vi "Asynchronous Engine.vi"(8 "error in":errorcluster, 9 "Parameters":T1, 10 "Parent":string) -> ()   [LabVIEW 2014, in "Waveform-Processing-Custom-Device Engine.lvlib"]
uses:
  Waveform-Processing-Custom-Device Engine.lvlib
  Types/Async Parameters.ctl
  Types/Async FIFOs.ctl
  <vilib>/NI Veristand/Custom Device Waveform API/Single Waveform Read (DBL)/Single Waveform Read (DBL).lvclass
  <userlib>/Circular Buffer/Controls/Circular Buffer Operations.ctl
  <userlib>/Circular Buffer/Instance VIs/Circular Buffer(2D DBL).vi
  Userlib/Error Handling API/Error Handling API.lvlib
  Userlib/Inline Async API/Inline Async API.lvlib
  <userlib>/Circular Buffer/Circular Buffer.lvlib
panel:
  out "Processing Engine Loop Rate (ms)":u32
  out "Tag Results":dbl[](array[numeric])
  in  "Stop":bool
  in  "Samples to average":i32=512
  out "error out":errorcluster
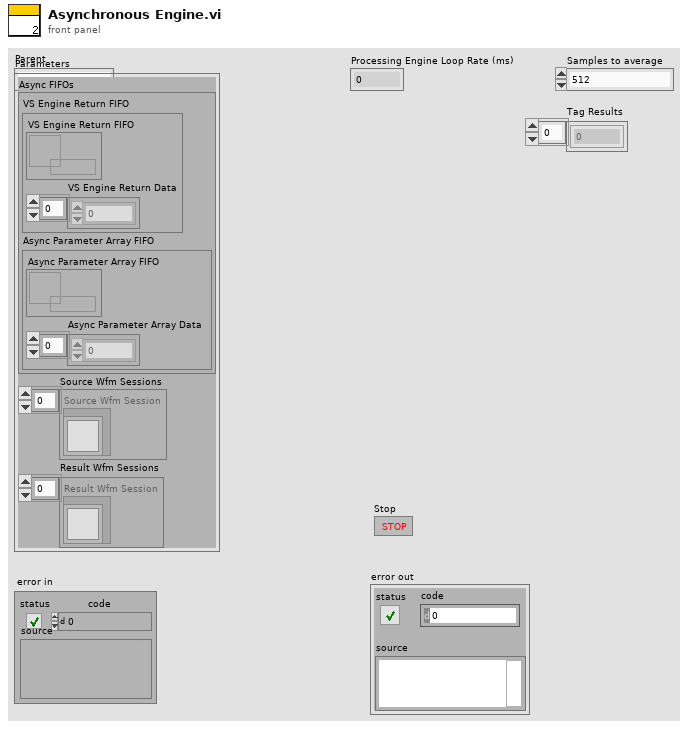
[diagram p1: front panel]
types:
  T1 = typedef "Waveform-Processing-Custom-Device Engine.lvlib/Async Parameters.ctl" = cluster{"Async FIFOs":T2, "Source Wfm Sessions":refnum<class "Single Waveform Read (DBL).lvclass">[], "Result Wfm Sessions":refnum<class "Single Waveform Read (DBL).lvclass">[]}
  T2 = typedef "Waveform-Processing-Custom-Device Engine.lvlib/Async FIFOs.ctl" = cluster{"VS Engine Return FIFO":cluster{"VS Engine Return FIFO":refnum<k33>, "VS Engine Return Data":dbl[]}, "Async Parameter Array FIFO":cluster{"Async Parameter Array FIFO":refnum<k33>, "Async Parameter Array Data":dbl[]}}
  T3 = cluster{"Samples per Channel":u32, "Channels":u32}
  T4 = typedef "Circular Buffer.lvlib/Circular Buffer Operations.ctl" = enum16{"Initialize", "Get Backlog", "Write", "Read (continuous)", "Read (most recent)"}
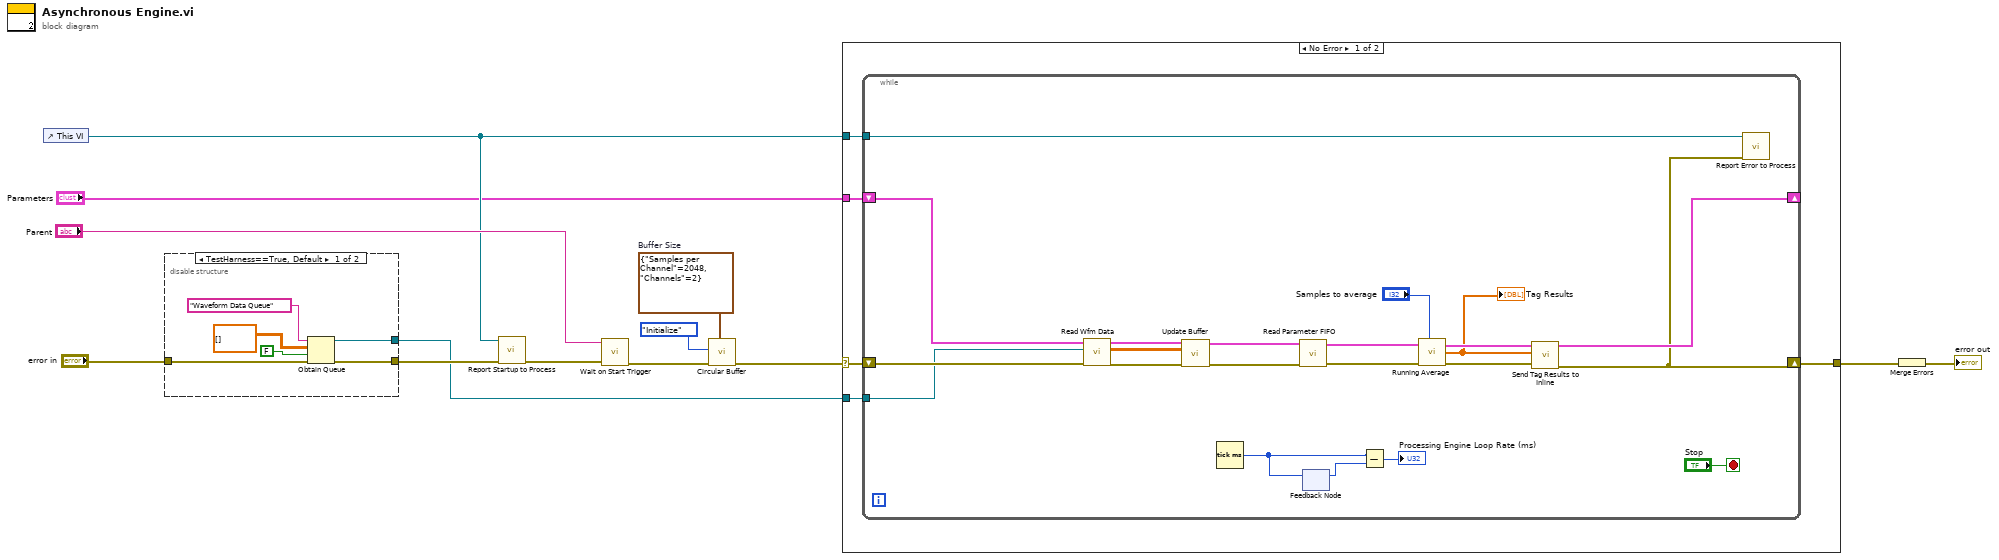
[diagram p0: block diagram]
diagram:
  w3 = T3 {"Samples per Channel"=2048, "Channels"=2}  # Buffer Size
  n1 = control-ref of="This VI"() -> (w11:refnum<vi>)
  n2 = disable-structure shown="TestHarness==True, Default" {
    disable-tunnel: [w16 _] -> w2
    disable-tunnel: [w15 _] -> w7
    disable-tunnel: "error in" -> [w14 _]
    frame condition #0 (active) {
      n3 = Obtain Queue(name (unnamed)="Waveform Data Queue", element data type=dbl[][] [], create if not found? (T)=FALSE, error in (no error)=w14) -> (queue out=w16:refnum<queue>, error out=w15:errorcluster)  [unwired: 1 in, 1 out]
    }
    frame condition #1 {
    }
  }
  n4 = call "Report Startup to Process.vi"("Error"=w7, "This VI"=w11) -> ("error out"=w13:errorcluster)  [unwired: 9 in]
  n5 = call "Wait on Start Trigger.vi"("error in (no error)"=w13, "Name"="Parent") -> ("error out"=w5:errorcluster)  [unwired: 8 in, 1 out]
  n6 = call-poly <userlib>:"Circular Buffer.vi"("Buffer Size"=w3, "error in (no error)"=w5, "Operation"=Circular_Buffer_Operations."Initialize") -> ("error out"=w4:errorcluster)  [unwired: 5 in, 3 out]
  n7 = case shown="No Error" w4 {
    selector: w4 -> [w24 _]
    tunnel: w11 -> [w23 _]
    tunnel: [w22 _] -> w10
    tunnel: w2 -> [w21 _]
    tunnel: "Parameters" -> [w20 _]
    frame No Error {
      n8 = while {
        shift-right: [w28] -> w22
        shift-left: w24 -> [w45]
        tunnel: w23 -> [w44]
        tunnel: w21 -> [w41]
        shift-right: [w29] -> _
        shift-left: w20 -> [w30]
        stop <- "Stop" stop-if-true
        n9 = call "Read Wfm Data.vi"("error in (no error)"=w45, "Queue in"=w41, "Parameters in"=w30) -> ("error out"=w38:errorcluster, "Wfm Data"=w36:dbl[][], "Parameters out"=w40:T1)  [unwired: 6 in]
        n10 = call "Update Buffer.vi"("Error in"=w38, "Wfm data"=w36, "Parameters"=w40) -> ("Error out"=w37:errorcluster, "Parameters dup"=w39:T1)  [unwired: 7 in]
        n11 = Tick Count (ms)() -> (millisecond timer value=w27:u32)
        n12 = call "Read Parameter FIFO.vi"("Error In"=w37, "Parameters in"=w39) -> ("Error Out"=w35:errorcluster, "Parameters out"=w34:T1)  [unwired: 8 in]
        n13 = feedback-in #1(w27) -> ()
        n14 = feedback #1() -> (w26:u32)  [unwired: 1 in]
        n15 = Subtract(x=w27, y=w26) -> (x-y=→"Processing Engine Loop Rate (ms)":u32)
        n16 = call "Running Average.vi"("Samples to average"="Samples to average", "Error In"=w35, "Parameters"=w34) -> ("Error Out"=w32:errorcluster, "Tag Results"=w31:dbl[], "Parameters dup"=w33:T1)  [unwired: 6 in]
        "Tag Results" <- w31
        n17 = call "Send Tag Results to Inline.vi"("Error in"=w32, "Tag Results"=w31, "Parameters"=w33) -> ("Error out"=w28:errorcluster, "Parameters dup"=w29:T1)  [unwired: 7 in]
        n18 = call "Report Error to Process.vi"("Error"=w28, "This VI"=w44) -> ()  [unwired: 10 in]
      }
    }
    frame Error {
    }
  }
  n19 = Merge Errors(w10) -> (→"error out":errorcluster)
